vi "Stop Core.vi"(10 "final error code":i32, 11 "Tracer-P in":refnum<class "Tracer-P.lvclass">) -> (3 "Tracer-P out":refnum<class "Tracer-P.lvclass">)   [LabVIEW 2013, in "Tracer-P.lvclass"]
doc: "(<B>Filename</B>: Actor Framework.lvlib:Actor.lvclass:Stop Core.vi)\n\nDefines what the actor does before it stops. Use the <B>final error code</B> input to determine whether the actor shut down in response to an error.\n\nBy default, this method does nothing. A descendant class may override it to define behavior, such as shutting down any processes the actor initiated in its override of the Actor Core method."
uses:
  Tracer-P.lvclass
  Logical Systems/Tracer/Tracer.lvclass
  Tracer-P.lvclass/Tracer-P.ctl
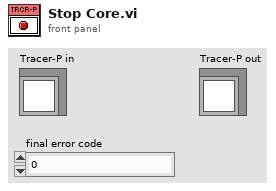
[diagram p1: front panel]
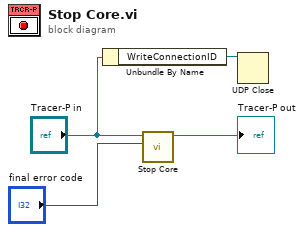
[diagram p0: block diagram]
diagram:
  n1 = Unbundle By Name("Tracer-P in") -> ("WriteConnectionID"=w1:refnum<k16>)
  n2 = call-parent "Stop Core.vi"("final error code"="final error code", "Actor in"="Tracer-P in") -> ("Actor out"=→"Tracer-P out":refnum<class "Tracer-P.lvclass">)  [unwired: 9 in]
  n3 = UDP Close(connection ID=w1) -> ()  [unwired: 1 in, 2 out]
